vi "TEST.vi"() -> ()   [LabVIEW 2021, in "LvMarkdown.lvlib"]
uses:
  LvMarkdown.lvlib
  LvMarkdown/Collection/Collection.lvclass
  C:/GitHub/LvMarkdown/src/LvMarkdown/IRenderable/IRenderable.lvclass
  LvMarkdown/Paragraph/Paragraph.lvclass
  C:/GitHub/LvMarkdown/src/LvMarkdown/Markdown.lvclass
  LvMarkdown/Line/Line.lvclass
  LvMarkdown/Blockquote/Blockquote.lvclass
  LvMarkdown/Heading/Heading.lvclass
  LvMarkdown/OrderedList/OrderedList.lvclass
  LvMarkdown/UnorderedList/UnorderedList.lvclass
  LvMarkdown/Image/Image.lvclass
  LvMarkdown/HorizontalRule/HorizontalRule.lvclass
  LvMarkdown/Url/Url.lvclass
  LvMarkdown/Link/Link.lvclass
  LvMarkdown/LineBreak/LineBreak.lvclass
  LvMarkdown/Bold/Bold.lvclass
  LvMarkdown/Italic/Italic.lvclass
  LvMarkdown/Table/Table.lvclass
  LvMarkdown/Code/Code.lvclass
  LvMarkdown/Alignment/AlignmentEnum.ctl
  LvMarkdown/Alignment/Alignment.lvclass
  LvMarkdown/FencedCodeBlock/FencedCodeBlock.lvclass
  LvMarkdown/Image/Image.lvclass/Image.ctl
  LvMarkdown/Heading/Heading.lvclass/Heading.ctl
  LvMarkdown/Link/Link.lvclass/Link.ctl
  LvMarkdown/Table/Table.lvclass/Table.ctl
  LvMarkdown/FencedCodeBlock/FencedCodeBlock.lvclass/FencedCodeBlock.ctl
  LvMarkdown/FencedCodeBlock/SetLanguage.vi
  LvMarkdown/Table/SetTableRow.vi
  LvMarkdown/Table/SetAlignment.vi
  LvMarkdown/Link/SetUrl.vi
  LvMarkdown/Image/SetTitle.vi
  LvMarkdown/Image/SetPath.vi
  LvMarkdown/Heading/SetHeadingLevel.vi
  LvMarkdown/OrderedList/SetOrderedList.vi
  LvMarkdown/UnorderedList/SetUnorderedList.vi
  LvMarkdown/Table/SetHeader.vi
  C:/GitHub/LvMarkdown/src/LvMarkdown/Heading/Heading.lvclass
  C:/GitHub/LvMarkdown/src/LvMarkdown/Paragraph/Paragraph.lvclass
  C:/GitHub/LvMarkdown/src/LvMarkdown/Line/Line.lvclass
  C:/GitHub/LvMarkdown/src/LvMarkdown/Italic/Italic.lvclass
  C:/GitHub/LvMarkdown/src/LvMarkdown/LineBreak/LineBreak.lvclass
  C:/GitHub/LvMarkdown/src/LvMarkdown/Blockquote/Blockquote.lvclass
  C:/GitHub/LvMarkdown/src/LvMarkdown/Collection/Collection.lvclass
  C:/GitHub/LvMarkdown/src/LvMarkdown/Bold/Bold.lvclass
  C:/GitHub/LvMarkdown/src/LvMarkdown/Code/Code.lvclass
  C:/GitHub/LvMarkdown/src/LvMarkdown/Link/Link.lvclass
  C:/GitHub/LvMarkdown/src/LvMarkdown/Table/Table.lvclass
  C:/GitHub/LvMarkdown/src/LvMarkdown/Image/Image.lvclass
  C:/GitHub/LvMarkdown/src/LvMarkdown/Url/Url.lvclass
  C:/GitHub/LvMarkdown/src/LvMarkdown/HorizontalRule/HorizontalRule.lvclass
  C:/GitHub/LvMarkdown/src/LvMarkdown/OrderedList/OrderedList.lvclass
  C:/GitHub/LvMarkdown/src/LvMarkdown/UnorderedList/UnorderedList.lvclass
  C:/GitHub/LvMarkdown/src/LvMarkdown/FencedCodeBlock/FencedCodeBlock.lvclass
panel:
  out "String out":string
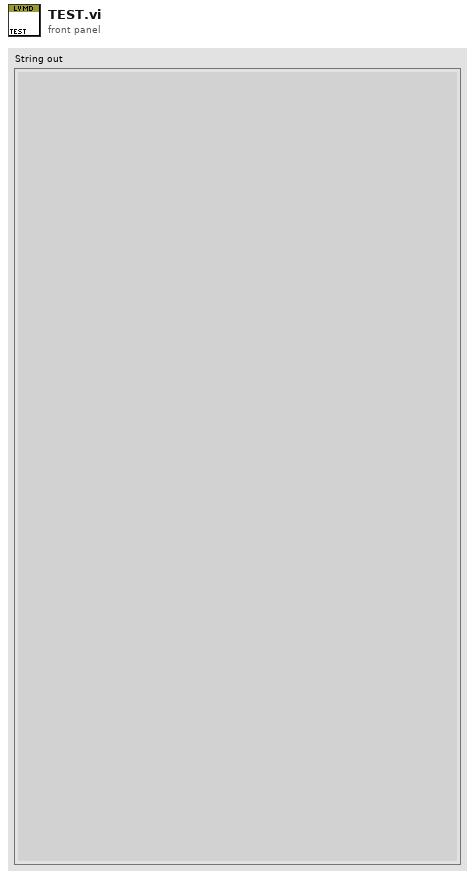
[diagram p1: front panel]
types:
  T1 = typedef "LvMarkdown.lvlib/Alignment.lvclass/AlignmentEnum.ctl" = enum16{"Left", "Center", "Right"}
  T2 = enum16{"Level 1", "Level 2", "Level 3", "Level 4", "Level 5", "Level 6"}
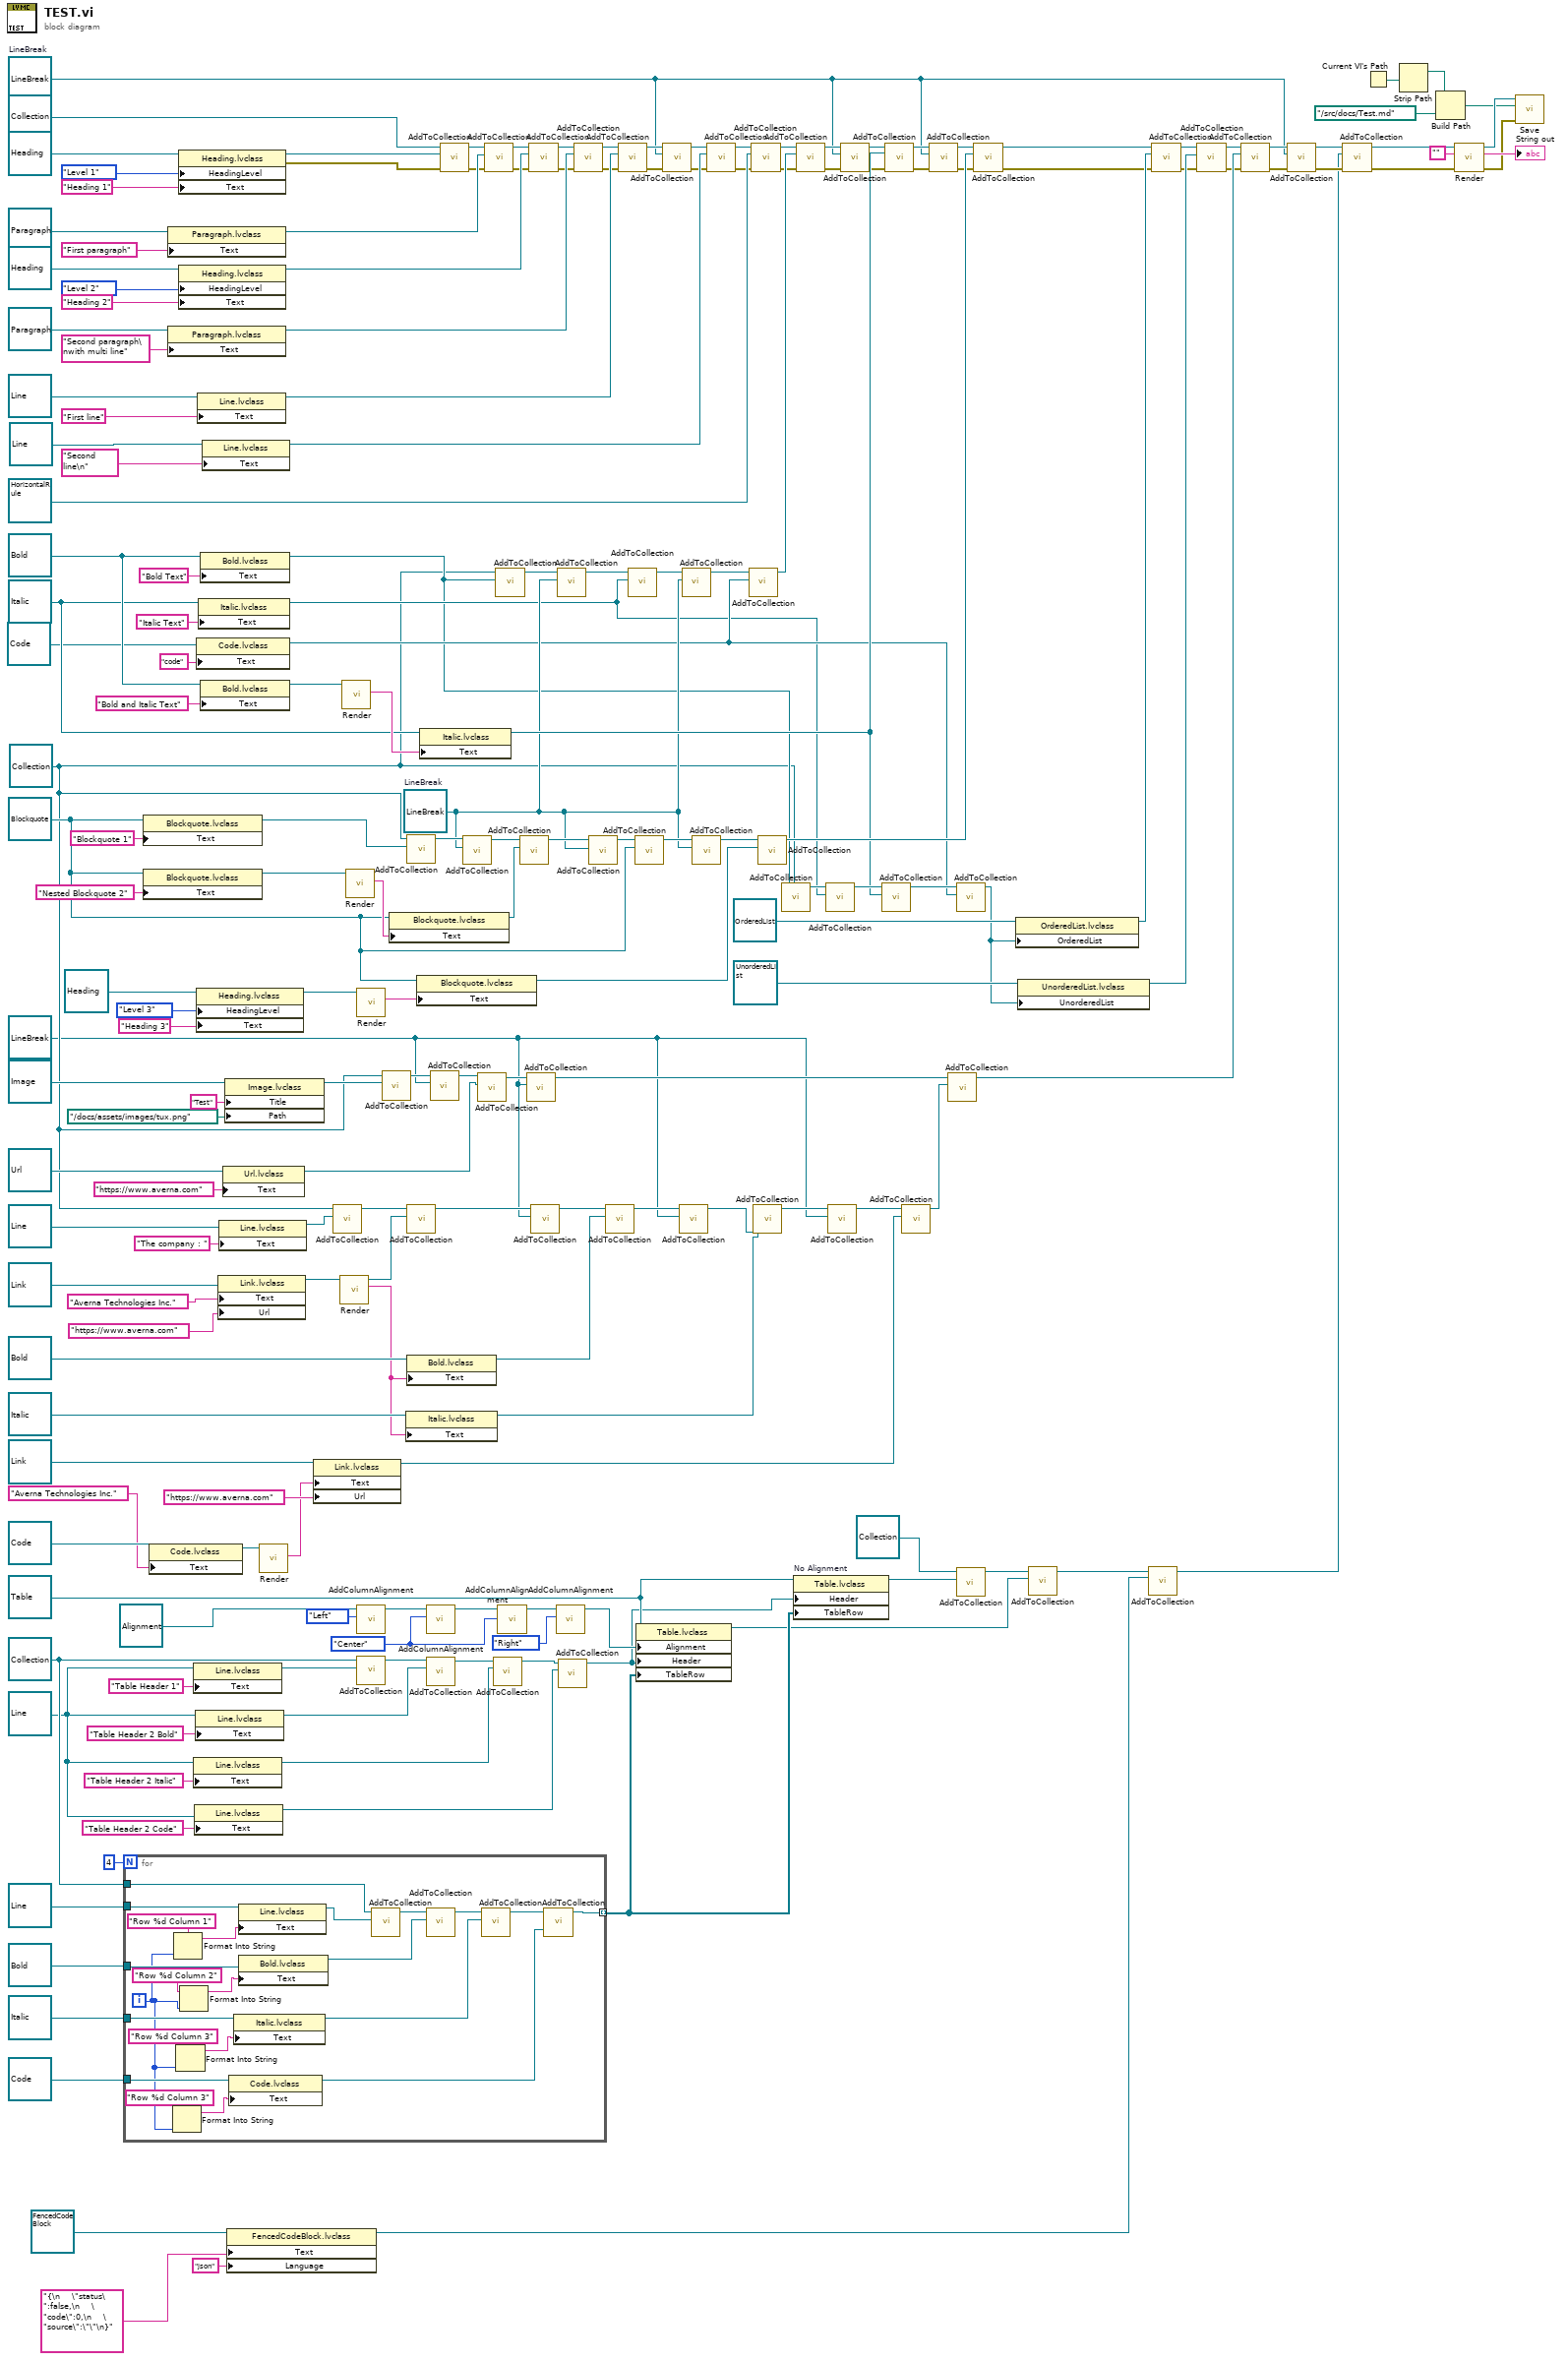
[diagram p0: block diagram]
diagram:
  w16 = AlignmentEnum."Center" ("Alignment")
  w41 = refnum<class "Collection.lvclass"> refnum ("Collection in")
  w26 = refnum<class "Line.lvclass"> refnum ("Markdown.lvlib:Line.lvclass")
  w13 = refnum<class "Table.lvclass"> refnum ("LvMarkdown.lvlib:Table.lvclass")
  w69 = refnum<class "LineBreak.lvclass"> refnum ("LineBreak")
  w111 = refnum<class "LineBreak.lvclass"> refnum  # LineBreak
  w89 = refnum<class "Collection.lvclass"> refnum ("Collection in")
  w133 = refnum<class "Blockquote.lvclass"> refnum ("Markdown.lvlib:Blockquote.lvclass")
  w161 = refnum<class "Italic.lvclass"> refnum ("Markdown.lvlib:Italic.lvclass")
  w165 = refnum<class "Bold.lvclass"> refnum ("Markdown.lvlib:Bold.lvclass")
  w33 = refnum<class "LineBreak.lvclass"> refnum  # LineBreak
  n1 = for {
    N: 4 -> [_]
    tunnel: refnum<class "Bold.lvclass"> refnum ("Markdown.lvlib:Bold.lvclass") -> [w214]
    tunnel: w41 -> [w216]
    tunnel: [w201] -> w12 mode=indexing
    tunnel: refnum<class "Line.lvclass"> refnum ("Markdown.lvlib:Line.lvclass") -> [w209]
    tunnel: refnum<class "Italic.lvclass"> refnum ("Markdown.lvlib:Italic.lvclass") -> [w207]
    tunnel: refnum<class "Code.lvclass"> refnum ("Markdown.lvlib:Code.lvclass") -> [w204]
    i -> [w199]
    n2 = Format Into String(format string="Row %d Column 3" ("Text"), w199) -> (resulting string=w203:string)  [unwired: 2 in, 1 out]
    n3 = Format Into String(format string="Row %d Column 1" ("Text"), w199) -> (resulting string=w213:string)  [unwired: 2 in, 1 out]
    n4 = Format Into String(format string="Row %d Column 3" ("Text"), w199) -> (resulting string=w208:string)  [unwired: 2 in, 1 out]
    n5 = Format Into String(format string="Row %d Column 2" ("Text"), w199) -> (resulting string=w212:string)  [unwired: 2 in, 1 out]
    n6 = property class="Code.lvclass"(reference=w204, "Text"=w203) -> (reference out=w200:refnum<class "Code.lvclass">)  [unwired: 1 in, 1 out]
    n7 = property class="Italic.lvclass"(reference=w207, "Text"=w208) -> (reference out=w205:refnum<class "Italic.lvclass">)  [unwired: 1 in, 1 out]
    n8 = property class="Line.lvclass"(reference=w209, "Text"=w213) -> (reference out=w217:refnum<class "Line.lvclass">)  [unwired: 1 in, 1 out]
    n9 = property class="Bold.lvclass"(reference=w214, "Text"=w212) -> (reference out=w215:refnum<class "Bold.lvclass">)  [unwired: 1 in, 1 out]
    n10 = call-dynamic "AddToCollection.vi"("IRenderable"=w217, "Collection in"=w216) -> ("Collection out"=w218:refnum<class "Collection.lvclass">)  [unwired: 8 in, 1 out]
    n11 = call-dynamic "AddToCollection.vi"("IRenderable"=w215, "Collection in"=w218) -> ("Collection out"=w206:refnum<class "Collection.lvclass">)  [unwired: 8 in, 1 out]
    n12 = call-dynamic "AddToCollection.vi"("IRenderable"=w205, "Collection in"=w206) -> ("Collection out"=w202:refnum<class "Collection.lvclass">)  [unwired: 8 in, 1 out]
    n13 = call-dynamic "AddToCollection.vi"("IRenderable"=w200, "Collection in"=w202) -> ("Collection out"=w201:refnum<class "Collection.lvclass">)  [unwired: 8 in, 1 out]
  }
  n14 = property class="Blockquote.lvclass"(reference=w133, "Text"="Blockquote 1") -> (reference out=w147:refnum<class "Blockquote.lvclass">)  [unwired: 1 in, 1 out]
  n15 = property class="Blockquote.lvclass"(reference=w133, "Text"="Nested Blockquote 2") -> (reference out=w145:refnum<class "Blockquote.lvclass">)  [unwired: 1 in, 1 out]
  n16 = property class="Code.lvclass"(reference=refnum<class "Code.lvclass"> refnum ("Markdown.lvlib:Code.lvclass"), "Text"="Averna Technologies Inc.") -> (reference out=w65:refnum<class "Code.lvclass">)  [unwired: 1 in, 1 out]
  n17 = property class="Paragraph.lvclass"(reference=refnum<class "Paragraph.lvclass"> refnum ("Markdown.lvlib:Paragraph.lvclass"), "Text"="First paragraph") -> (reference out=w183:refnum<class "Paragraph.lvclass">)  [unwired: 1 in, 1 out]
  n18 = property class="Paragraph.lvclass"(reference=refnum<class "Paragraph.lvclass"> refnum ("Markdown.lvlib:Paragraph.lvclass"), "Text"="Second paragraph\nwith multi line") -> (reference out=w177:refnum<class "Paragraph.lvclass">)  [unwired: 1 in, 1 out]
  n19 = property class="Heading.lvclass"(reference=refnum<class "Heading.lvclass"> refnum ("Markdown.lvlib:Heading.lvclass"), "HeadingLevel"=T2."Level 1", "Text"="Heading 1") -> (reference out=w192:refnum<class "Heading.lvclass">, error out=w47:errorcluster)  [unwired: 1 in]
  n20 = property class="Heading.lvclass"(reference=refnum<class "Heading.lvclass"> refnum ("Markdown.lvlib:Heading.lvclass"), "HeadingLevel"=T2."Level 2" ("HeadingLevel 2"), "Text"="Heading 2") -> (reference out=w182:refnum<class "Heading.lvclass">)  [unwired: 1 in, 1 out]
  n21 = property class="Line.lvclass"(reference=w26, "Text"="Table Header 1") -> (reference out=w43:refnum<class "Line.lvclass">)  [unwired: 1 in, 1 out]
  n22 = property class="Line.lvclass"(reference=w26, "Text"="Table Header 2 Italic") -> (reference out=w23:refnum<class "Line.lvclass">)  [unwired: 1 in, 1 out]
  n23 = property class="Line.lvclass"(reference=w26, "Text"="Table Header 2 Code") -> (reference out=w22:refnum<class "Line.lvclass">)  [unwired: 1 in, 1 out]
  n24 = property class="Line.lvclass"(reference=w26, "Text"="Table Header 2 Bold") -> (reference out=w44:refnum<class "Line.lvclass">)  [unwired: 1 in, 1 out]
  n25 = property class="Code.lvclass"(reference=refnum<class "Code.lvclass"> refnum ("Markdown.lvlib:Code.lvclass"), "Text"="code") -> (reference out=w107:refnum<class "Code.lvclass">)  [unwired: 1 in, 1 out]
  n26 = property class="Heading.lvclass"(reference=refnum<class "Heading.lvclass"> refnum ("Markdown.lvlib:Heading.lvclass"), "HeadingLevel"=T2."Level 3", "Text"="Heading 3") -> (reference out=w137:refnum<class "Heading.lvclass">)  [unwired: 1 in, 1 out]
  n27 = property class="Line.lvclass"(reference=refnum<class "Line.lvclass"> refnum ("Markdown.lvlib:Line.lvclass"), "Text"="First line") -> (reference out=w171:refnum<class "Line.lvclass">)  [unwired: 1 in, 1 out]
  n28 = property class="Italic.lvclass"(reference=w161, "Text"="Italic Text") -> (reference out=w106:refnum<class "Italic.lvclass">)  [unwired: 1 in, 1 out]
  n29 = property class="Bold.lvclass"(reference=w165, "Text"="Bold Text") -> (reference out=w105:refnum<class "Bold.lvclass">)  [unwired: 1 in, 1 out]
  n30 = property class="Bold.lvclass"(reference=w165, "Text"="Bold and Italic Text") -> (reference out=w164:refnum<class "Bold.lvclass">)  [unwired: 1 in, 1 out]
  n31 = property class="Line.lvclass"(reference=refnum<class "Line.lvclass"> refnum ("Markdown.lvlib:Line.lvclass"), "Text"="Second line\n") -> (reference out=w168:refnum<class "Line.lvclass">)  [unwired: 1 in, 1 out]
  n32 = property class="Link.lvclass"(reference=refnum<class "Link.lvclass"> refnum ("Markdown.lvlib:Link.lvclass"), "Text"="Averna Technologies Inc.", "Url"="https://www.averna.com" ("Text")) -> (reference out=w90:refnum<class "Link.lvclass">)  [unwired: 1 in, 1 out]
  n33 = property class="Line.lvclass"(reference=refnum<class "Line.lvclass"> refnum ("Markdown.lvlib:Line.lvclass"), "Text"="The company : ") -> (reference out=w85:refnum<class "Line.lvclass">)  [unwired: 1 in, 1 out]
  n34 = property class="Url.lvclass"(reference=refnum<class "Url.lvclass"> refnum ("Markdown.lvlib:Url.lvclass"), "Text"="https://www.averna.com") -> (reference out=w100:refnum<class "Url.lvclass">)  [unwired: 1 in, 1 out]
  n35 = property class="Image.lvclass"(reference=refnum<class "Image.lvclass"> refnum ("Markdown.lvlib:Image.lvclass"), "Title"="Test", "Path"=path "../docs/assets/images/tux.png") -> (reference out=w101:refnum<class "Image.lvclass">)  [unwired: 1 in, 1 out]
  n36 = property class="FencedCodeBlock.lvclass"(reference=refnum<class "FencedCodeBlock.lvclass"> refnum ("LvMarkdown.lvlib:FencedCodeBlock.lvclass"), "Text"="{\n    \"status\":false,\n    \"code\":0,\n    \"source\":\"\"\n}", "Language"="json") -> (reference out=w4:refnum<class "FencedCodeBlock.lvclass">)  [unwired: 1 in, 1 out]
  n37 = call-dynamic "Render.vi"("Bold in"=w65) -> ("String out"=w64:string)  [unwired: 8 in, 2 out]
  n38 = property class="Link.lvclass"(reference=refnum<class "Link.lvclass"> refnum ("Markdown.lvlib:Link.lvclass"), "Text"=w64, "Url"="https://www.averna.com" ("Text")) -> (reference out=w68:refnum<class "Link.lvclass">)  [unwired: 1 in, 1 out]
  n39 = call-dynamic "AddToCollection.vi"("IRenderable"=w85, "Collection in"=w89) -> ("Collection out"=w88:refnum<class "Collection.lvclass">)  [unwired: 8 in, 1 out]
  n40 = call-dynamic "Render.vi"("Link in"=w90) -> ("String out"=w77:string, "Link out"=w84:refnum<class "Link.lvclass">)  [unwired: 8 in, 1 out]
  n41 = call-dynamic "Render.vi"("Bold in"=w164) -> ("String out"=w163:string)  [unwired: 8 in, 2 out]
  n42 = call-dynamic "Render.vi"("Blockquote in"=w145) -> ("String out"=w144:string)  [unwired: 8 in, 2 out]
  n43 = call-dynamic "Render.vi"("Heading in"=w137) -> ("String out"=w136:string)  [unwired: 8 in, 2 out]
  n44 = call "AddColumnAlignment.vi"("Alignment"=AlignmentEnum."Left", "Alignment in"=refnum<class "Alignment.lvclass"> refnum ("LvMarkdown.lvlib:Alignment.lvclass")) -> ("Alignment out"=w21:refnum<class "Alignment.lvclass">)  [unwired: 8 in, 1 out]
  n45 = call-dynamic "AddToCollection.vi"("IRenderable"=w43, "Collection in"=w41) -> ("Collection out"=w42:refnum<class "Collection.lvclass">)  [unwired: 8 in, 1 out]
  n46 = call-dynamic "AddToCollection.vi"("IRenderable"=w101, "Collection in"=w89) -> ("Collection out"=w94:refnum<class "Collection.lvclass">)  [unwired: 8 in, 1 out]
  n47 = property class="Blockquote.lvclass"(reference=w133, "Text"=w144) -> (reference out=w143:refnum<class "Blockquote.lvclass">)  [unwired: 1 in, 1 out]
  n48 = property class="Italic.lvclass"(reference=refnum<class "Italic.lvclass"> refnum ("Markdown.lvlib:Italic.lvclass"), "Text"=w77) -> (reference out=w75:refnum<class "Italic.lvclass">)  [unwired: 1 in, 1 out]
  n49 = call-dynamic "AddToCollection.vi"("IRenderable"=w147, "Collection in"=w89) -> ("Collection out"=w148:refnum<class "Collection.lvclass">)  [unwired: 8 in, 1 out]
  n50 = call-dynamic "AddToCollection.vi"("IRenderable"=w84, "Collection in"=w88) -> ("Collection out"=w80:refnum<class "Collection.lvclass">)  [unwired: 8 in, 1 out]
  n51 = property class="Bold.lvclass"(reference=refnum<class "Bold.lvclass"> refnum ("Markdown.lvlib:Bold.lvclass"), "Text"=w77) -> (reference out=w79:refnum<class "Bold.lvclass">)  [unwired: 1 in, 1 out]
  n52 = property class="Blockquote.lvclass"(reference=w133, "Text"=w136) -> (reference out=w135:refnum<class "Blockquote.lvclass">)  [unwired: 1 in, 1 out]
  n53 = property class="Italic.lvclass"(reference=w161, "Text"=w163) -> (reference out=w126:refnum<class "Italic.lvclass">)  [unwired: 1 in, 1 out]
  n54 = call "AddColumnAlignment.vi"("Alignment"=w16, "Alignment in"=w21) -> ("Alignment out"=w20:refnum<class "Alignment.lvclass">)  [unwired: 8 in, 1 out]
  n55 = call-dynamic "AddToCollection.vi"("IRenderable"=w44, "Collection in"=w42) -> ("Collection out"=w24:refnum<class "Collection.lvclass">)  [unwired: 8 in, 1 out]
  n56 = call-dynamic "AddToCollection.vi"("IRenderable"=w69, "Collection in"=w94) -> ("Collection out"=w93:refnum<class "Collection.lvclass">)  [unwired: 8 in, 1 out]
  n57 = call-dynamic "AddToCollection.vi"("error in (no error)"=w47, "IRenderable"=w192, "Collection in"=refnum<class "Collection.lvclass"> refnum ("Markdown.lvlib:Collection.lvclass")) -> ("error out"=w63:errorcluster, "Collection out"=w186:refnum<class "Collection.lvclass">)  [unwired: 7 in]
  n58 = call-dynamic "AddToCollection.vi"("IRenderable"=w111, "Collection in"=w148) -> ("Collection out"=w146:refnum<class "Collection.lvclass">)  [unwired: 8 in, 1 out]
  n59 = call-dynamic "AddToCollection.vi"("IRenderable"=w100, "Collection in"=w93) -> ("Collection out"=w92:refnum<class "Collection.lvclass">)  [unwired: 8 in, 1 out]
  n60 = call-dynamic "AddToCollection.vi"("error in (no error)"=w63, "IRenderable"=w183, "Collection in"=w186) -> ("error out"=w62:errorcluster, "Collection out"=w184:refnum<class "Collection.lvclass">)  [unwired: 7 in]
  n61 = call-dynamic "AddToCollection.vi"("IRenderable"=w23, "Collection in"=w24) -> ("Collection out"=w25:refnum<class "Collection.lvclass">)  [unwired: 8 in, 1 out]
  n62 = call-dynamic "AddToCollection.vi"("IRenderable"=w105, "Collection in"=w89) -> ("Collection out"=w113:refnum<class "Collection.lvclass">)  [unwired: 8 in, 1 out]
  n63 = call "AddColumnAlignment.vi"("Alignment"=w16, "Alignment in"=w20) -> ("Alignment out"=w19:refnum<class "Alignment.lvclass">)  [unwired: 8 in, 1 out]
  n64 = call-dynamic "AddToCollection.vi"("IRenderable"=w143, "Collection in"=w146) -> ("Collection out"=w142:refnum<class "Collection.lvclass">)  [unwired: 8 in, 1 out]
  n65 = call-dynamic "AddToCollection.vi"("IRenderable"=w69, "Collection in"=w92) -> ("Collection out"=w91:refnum<class "Collection.lvclass">)  [unwired: 8 in, 1 out]
  n66 = call-dynamic "AddToCollection.vi"("error in (no error)"=w62, "IRenderable"=w182, "Collection in"=w184) -> ("error out"=w61:errorcluster, "Collection out"=w178:refnum<class "Collection.lvclass">)  [unwired: 7 in]
  n67 = call-dynamic "AddToCollection.vi"("IRenderable"=w69, "Collection in"=w80) -> ("Collection out"=w82:refnum<class "Collection.lvclass">)  [unwired: 8 in, 1 out]
  n68 = call "AddColumnAlignment.vi"("Alignment"=AlignmentEnum."Right", "Alignment in"=w19) -> ("Alignment out"=w18:refnum<class "Alignment.lvclass">)  [unwired: 8 in, 1 out]
  n69 = call-dynamic "AddToCollection.vi"("IRenderable"=w111, "Collection in"=w113) -> ("Collection out"=w112:refnum<class "Collection.lvclass">)  [unwired: 8 in, 1 out]
  n70 = call-dynamic "AddToCollection.vi"("IRenderable"=w22, "Collection in"=w25) -> ("Collection out"=w11:refnum<class "Collection.lvclass">)  [unwired: 8 in, 1 out]
  n71 = call-dynamic "AddToCollection.vi"("error in (no error)"=w61, "IRenderable"=w177, "Collection in"=w178) -> ("error out"=w60:errorcluster, "Collection out"=w172:refnum<class "Collection.lvclass">)  [unwired: 7 in]
  n72 = call-dynamic "AddToCollection.vi"("IRenderable"=w111, "Collection in"=w142) -> ("Collection out"=w134:refnum<class "Collection.lvclass">)  [unwired: 8 in, 1 out]
  n73 = call-dynamic "AddToCollection.vi"("IRenderable"=w79, "Collection in"=w82) -> ("Collection out"=w81:refnum<class "Collection.lvclass">)  [unwired: 8 in, 1 out]
  n74 = call-dynamic "AddToCollection.vi"("error in (no error)"=w60, "IRenderable"=w171, "Collection in"=w172) -> ("error out"=w59:errorcluster, "Collection out"=w170:refnum<class "Collection.lvclass">)  [unwired: 7 in]
  n75 = call-dynamic "AddToCollection.vi"("IRenderable"=w106, "Collection in"=w112) -> ("Collection out"=w115:refnum<class "Collection.lvclass">)  [unwired: 8 in, 1 out]
  n76 = call-dynamic "AddToCollection.vi"("IRenderable"=w133, "Collection in"=w134) -> ("Collection out"=w132:refnum<class "Collection.lvclass">)  [unwired: 8 in, 1 out]
  n77 = property class="Table.lvclass"(reference=w13, "Alignment"=w18, "Header"=w11, "TableRow"=w12) -> (reference out=w9:refnum<class "Table.lvclass">)  [unwired: 1 in, 1 out]
  n78 = call-dynamic "AddToCollection.vi"("error in (no error)"=w59, "IRenderable"=w33, "Collection in"=w170) -> ("error out"=w58:errorcluster, "Collection out"=w169:refnum<class "Collection.lvclass">)  [unwired: 7 in]
  n79 = call-dynamic "AddToCollection.vi"("IRenderable"=w69, "Collection in"=w81) -> ("Collection out"=w76:refnum<class "Collection.lvclass">)  [unwired: 8 in, 1 out]
  n80 = call-dynamic "AddToCollection.vi"("IRenderable"=w111, "Collection in"=w115) -> ("Collection out"=w114:refnum<class "Collection.lvclass">)  [unwired: 8 in, 1 out]
  n81 = call-dynamic "AddToCollection.vi"("IRenderable"=w111, "Collection in"=w132) -> ("Collection out"=w131:refnum<class "Collection.lvclass">)  [unwired: 8 in, 1 out]
  n82 = call-dynamic "AddToCollection.vi"("error in (no error)"=w58, "IRenderable"=w168, "Collection in"=w169) -> ("error out"=w57:errorcluster, "Collection out"=w155:refnum<class "Collection.lvclass">)  [unwired: 7 in]
  n83 = call-dynamic "AddToCollection.vi"("IRenderable"=w107, "Collection in"=w114) -> ("Collection out"=w116:refnum<class "Collection.lvclass">)  [unwired: 8 in, 1 out]
  n84 = call-dynamic "AddToCollection.vi"("error in (no error)"=w57, "IRenderable"=refnum<class "HorizontalRule.lvclass"> refnum ("Markdown.lvlib:HorizontalRule.lvclass"), "Collection in"=w155) -> ("error out"=w56:errorcluster, "Collection out"=w104:refnum<class "Collection.lvclass">)  [unwired: 7 in]
  n85 = call-dynamic "AddToCollection.vi"("IRenderable"=w75, "Collection in"=w76) -> ("Collection out"=w71:refnum<class "Collection.lvclass">)  [unwired: 8 in, 1 out]
  n86 = call-dynamic "AddToCollection.vi"("IRenderable"=w135, "Collection in"=w131) -> ("Collection out"=w141:refnum<class "Collection.lvclass">)  [unwired: 8 in, 1 out]
  n87 = call-dynamic "AddToCollection.vi"("IRenderable"=w105, "Collection in"=w89) -> ("Collection out"=w110:refnum<class "Collection.lvclass">)  [unwired: 8 in, 1 out]
  n88 = property on="No Alignment" class="Table.lvclass"(reference=w13, "Header"=w11, "TableRow"=w12) -> (reference out=w8:refnum<class "Table.lvclass">)  [unwired: 1 in, 1 out]
  n89 = call-dynamic "AddToCollection.vi"("error in (no error)"=w56, "IRenderable"=w116, "Collection in"=w104) -> ("error out"=w55:errorcluster, "Collection out"=w154:refnum<class "Collection.lvclass">)  [unwired: 7 in]
  n90 = call-dynamic "AddToCollection.vi"("IRenderable"=w106, "Collection in"=w110) -> ("Collection out"=w127:refnum<class "Collection.lvclass">)  [unwired: 8 in, 1 out]
  n91 = call-dynamic "AddToCollection.vi"("IRenderable"=w69, "Collection in"=w71) -> ("Collection out"=w72:refnum<class "Collection.lvclass">)  [unwired: 8 in, 1 out]
  n92 = call-dynamic "AddToCollection.vi"("error in (no error)"=w55, "IRenderable"=w33, "Collection in"=w154) -> ("error out"=w54:errorcluster, "Collection out"=w153:refnum<class "Collection.lvclass">)  [unwired: 7 in]
  n93 = call-dynamic "AddToCollection.vi"("IRenderable"=w126, "Collection in"=w127) -> ("Collection out"=w109:refnum<class "Collection.lvclass">)  [unwired: 8 in, 1 out]
  n94 = call-dynamic "AddToCollection.vi"("error in (no error)"=w54, "IRenderable"=w126, "Collection in"=w153) -> ("error out"=w53:errorcluster, "Collection out"=w152:refnum<class "Collection.lvclass">)  [unwired: 7 in]
  n95 = call-dynamic "AddToCollection.vi"("IRenderable"=w68, "Collection in"=w72) -> ("Collection out"=w70:refnum<class "Collection.lvclass">)  [unwired: 8 in, 1 out]
  n96 = call-dynamic "AddToCollection.vi"("error in (no error)"=w53, "IRenderable"=w33, "Collection in"=w152) -> ("error out"=w52:errorcluster, "Collection out"=w150:refnum<class "Collection.lvclass">)  [unwired: 7 in]
  n97 = call-dynamic "AddToCollection.vi"("IRenderable"=w70, "Collection in"=w91) -> ("Collection out"=w95:refnum<class "Collection.lvclass">)  [unwired: 8 in, 1 out]
  n98 = call-dynamic "AddToCollection.vi"("IRenderable"=w107, "Collection in"=w109) -> ("Collection out"=w108:refnum<class "Collection.lvclass">)  [unwired: 8 in, 1 out]
  n99 = call-dynamic "AddToCollection.vi"("IRenderable"=w8, "Collection in"=refnum<class "Collection.lvclass"> refnum) -> ("Collection out"=w10:refnum<class "Collection.lvclass">)  [unwired: 8 in, 1 out]
  n100 = call-dynamic "AddToCollection.vi"("error in (no error)"=w52, "IRenderable"=w141, "Collection in"=w150) -> ("error out"=w51:errorcluster, "Collection out"=w128:refnum<class "Collection.lvclass">)  [unwired: 7 in]
  n101 = property class="OrderedList.lvclass"(reference=refnum<class "OrderedList.lvclass"> refnum ("Markdown.lvlib:OrderedList.lvclass"), "OrderedList"=w108) -> (reference out=w129:refnum<class "OrderedList.lvclass">)  [unwired: 1 in, 1 out]
  n102 = property class="UnorderedList.lvclass"(reference=refnum<class "UnorderedList.lvclass"> refnum ("Markdown.lvlib:UnorderedList.lvclass"), "UnorderedList"=w108) -> (reference out=w124:refnum<class "UnorderedList.lvclass">)  [unwired: 1 in, 1 out]
  n103 = call-dynamic "AddToCollection.vi"("IRenderable"=w9, "Collection in"=w10) -> ("Collection out"=w1:refnum<class "Collection.lvclass">)  [unwired: 8 in, 1 out]
  n104 = call-dynamic "AddToCollection.vi"("IRenderable"=w4, "Collection in"=w1) -> ("Collection out"=w6:refnum<class "Collection.lvclass">)  [unwired: 8 in, 1 out]
  n105 = call-dynamic "AddToCollection.vi"("error in (no error)"=w51, "IRenderable"=w129, "Collection in"=w128) -> ("error out"=w50:errorcluster, "Collection out"=w123:refnum<class "Collection.lvclass">)  [unwired: 7 in]
  n106 = call-dynamic "AddToCollection.vi"("error in (no error)"=w50, "IRenderable"=w124, "Collection in"=w123) -> ("error out"=w49:errorcluster, "Collection out"=w120:refnum<class "Collection.lvclass">)  [unwired: 7 in]
  n107 = call-dynamic "AddToCollection.vi"("error in (no error)"=w49, "IRenderable"=w95, "Collection in"=w120) -> ("error out"=w37:errorcluster, "Collection out"=w35:refnum<class "Collection.lvclass">)  [unwired: 7 in]
  n108 = call-dynamic "AddToCollection.vi"("error in (no error)"=w37, "IRenderable"=w33, "Collection in"=w35) -> ("error out"=w36:errorcluster, "Collection out"=w34:refnum<class "Collection.lvclass">)  [unwired: 7 in]
  n109 = call-dynamic "AddToCollection.vi"("error in (no error)"=w36, "IRenderable"=w6, "Collection in"=w34) -> ("error out"=w39:errorcluster, "Collection out"=w38:refnum<class "Collection.lvclass">)  [unwired: 7 in]
  n110 = Current VI's Path() -> (path=w159:path)
  n111 = Strip Path(path=w159) -> (stripped path=w158:path)  [unwired: 1 out]
  n112 = Build Path(base path=w158, name or relative path=path "../src/docs/Test.md") -> (appended path=w157:path)
  n113 = call-dynamic "Render.vi"("error in (no error)"=w39, "String in"="", "Collection in"=w38) -> ("error out"=w48:errorcluster, "String out"=→"String out":string, "Collection out"=w160:refnum<class "Collection.lvclass">)  [unwired: 6 in]
  n114 = call "Save.vi"("error in (no error)"=w48, "Path"=w157, "Collection in"=w160) -> ()  [unwired: 7 in, 2 out]
